vi "Load.vi"(8 "Error In":errorcluster, 10 "Key":string, 11 "Loader In":refnum<class "File.lvclass">) -> (0 "Error Out":errorcluster, 2 "Template":string, 3 "Loader Out":refnum<class "File.lvclass">)   [LabVIEW 2018, in "Toolkit.lvlib" / "Loaders.lvlib" / "File.lvclass"]
doc: "Gets a template as a string based on the Partial's key value in the root, or master, template.\n\n<B>Loader In/Out</B> - Represents an implementation capable of loading, or including, a partial Mustache template.\n\n<B>Key</B> - The key from the partial tag.\n\n<B>Template</B> - The partial Mustache template associated with the key. The origin of the template depends on the loader's implementation and the data type associated with the key."
uses:
  File.lvclass
  File.lvclass/File.ctl
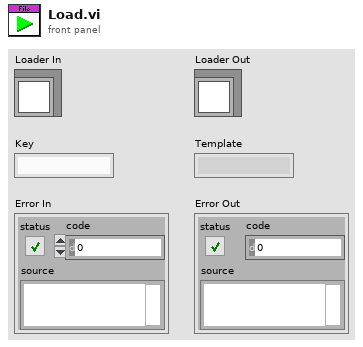
[diagram p1: front panel]
types:
  T1 = enum16{"open", "replace", "create", "open or create", "replace or create", "replace or create with confirmation"}
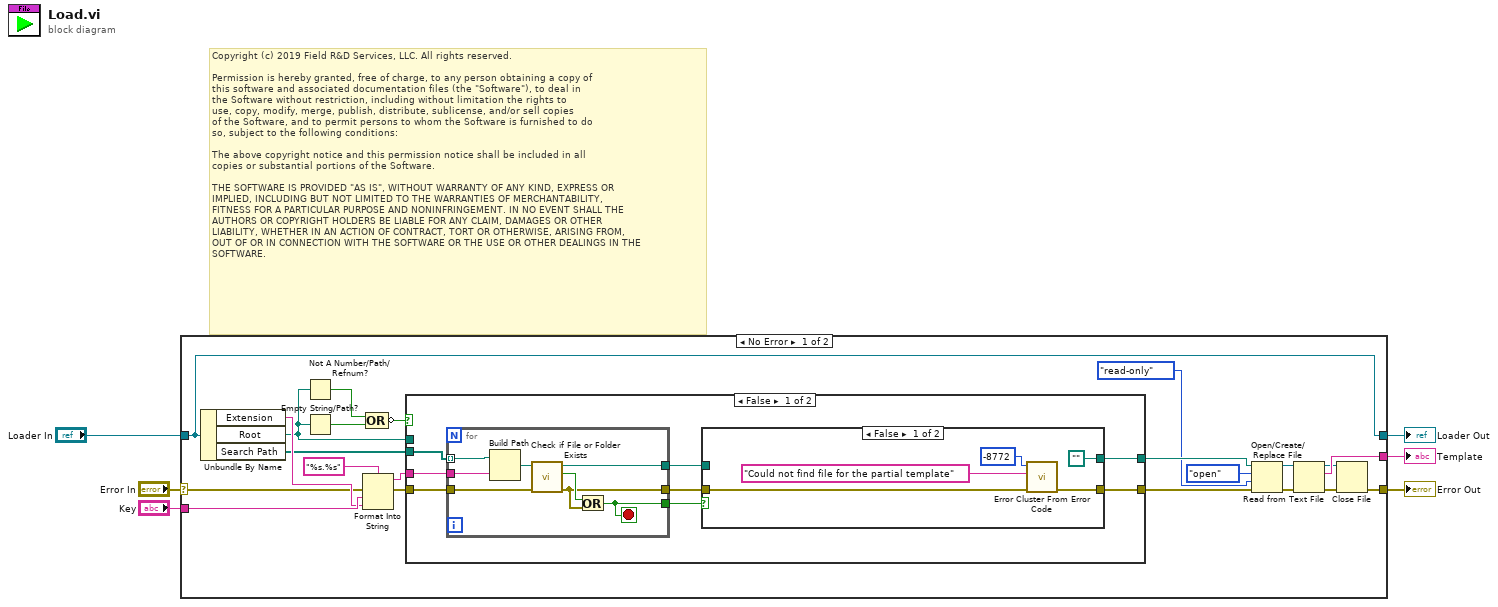
[diagram p0: block diagram]
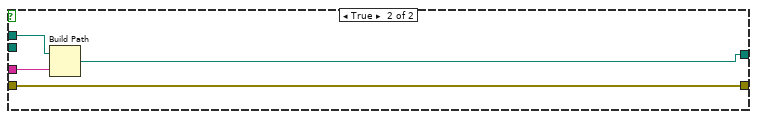
[diagram p3: hidden frame]
diagram:
  # "Copyright (c) 2019 Field R&D Services, LLC. All rights reserved.\n\nPermission is hereby granted, free of charge, to any person obtaining a copy of\nthis software and associated documentation files (the \"Software\"), to deal in\nthe Software without restriction, including without limitation the rights to\nuse, copy, modify, merge, publish, distribute, sublicense, and/or sell copies\nof the Software, and to permit persons to whom the Software is furnished to do\nso, subject to the following conditions:\n\nThe above copyright notice and this permission notice shall be included in all\ncopies or substantial portions of the Software.\n\nTHE SOFTWARE IS PROVIDED \"AS IS\", WITHOUT WARRANTY OF ANY KIND, EXPRESS OR\nIMPLIED, INCLUDING BUT NOT LIMITED TO THE WARRANTIES OF MERCHANTABILITY,\nFITNESS FOR A PARTICULAR PURPOSE AND NONINFRINGEMENT. IN NO EVENT SHALL THE\nAUTHORS OR COPYRIGHT HOLDERS BE LIABLE FOR ANY CLAIM, DAMAGES OR OTHER\nLIABILITY, WHETHER IN AN ACTION OF CONTRACT, TORT OR OTHERWISE, ARISING FROM,\nOUT OF OR IN CONNECTION WITH THE SOFTWARE OR THE USE OR OTHER DEALINGS IN THE\nSOFTWARE."
  n1 = case shown="No Error" "Error In" {
    selector: "Error In" -> [w25 w57]
    tunnel: [w16 w57] -> w5
    tunnel: "Loader In" -> [w15 w56]
    tunnel: [w15 w56] -> w3
    tunnel: "Key" -> [w28 _]
    tunnel: [w13 _] -> w1
    frame No Error {
      n2 = Unbundle By Name(w15) -> ("Extension"=w26:string, "Root"=w20:path, "Search Path"=w18:path[])
      n3 = Not A Number/Path/Refnum?(number/path/refnum=w20) -> (NaN/Path/Refnum?=w23:bool)
      n4 = Empty String/Path?(string/path=w20) -> (empty?=w24:bool)
      n5 = Format Into String(format string="%s.%s", error in=w25, w28, w26) -> (resulting string=w21:string, error out=w19:errorcluster)  [unwired: 1 in]
      n6 = Compound Arithmetic op=OR(w23, w24) -> (invert w22:bool)
      n7 = case shown="False" w22 {
        tunnel: w21 -> [w30 w55]
        tunnel: w20 -> [_ w54]
        tunnel: [w33 w53] -> w14
        tunnel: w19 -> [w36 w52]
        tunnel: [w31 w52] -> w17
        tunnel: w18 -> [w29 _]
        frame False {
          n8 = for {
            tunnel: w29 -> [w46] mode=indexing
            tunnel: w36 -> [w51]
            tunnel: [w49] -> w32
            tunnel: [w48] -> w34
            tunnel: [w47] -> w35
            tunnel: w30 -> [w45]
            stop <- w47 stop-if-true
            n9 = Build Path(base path=w46, name or relative path=w45) -> (appended path=w44:path)
            n10 = call <vilib>:"Check if File or Folder Exists.vi"("error in (no error)"=w51, "path"=w44) -> ("error out"=w49:errorcluster, "file or folder exists?"=w50:bool, "dup path"=w48:path)  [unwired: 7 in]
            n11 = Or(x=w50, y=w49) -> (x .or. y?=w47:bool)
          }
          n12 = case shown="False" w35 {
            tunnel: w34 -> [_ w43]
            tunnel: [path "" w43] -> w33
            tunnel: w32 -> [w40 w42]
            tunnel: [w39 w42] -> w31
            frame False {
              n13 = call <vilib>:"Error Cluster From Error Code.vi"("error in (no error)"=w40, "error message (\"\")"="Could not find file for the partial template" ("error message (\"\")"), "error code (0)"=-8772) -> ("error out"=w39:errorcluster)  [unwired: 6 in]
            }
            frame True {
            }
          }
        }
        frame True {
          n14 = Build Path(base path=w54, name or relative path=w55) -> (appended path=w53:path)
        }
      }
      n15 = Open/Create/Replace File(file path (use dialog)=w14, error in=w17, operation (0:open)=T1."open", access (0:read/write)=enum16{"read/write", "read-only", "write-only"}."read-only") -> (refnum out=w10:refnum<file>, error out=w9:errorcluster)  [unwired: 2 in, 1 out]
      n16 = Read from Text File(file (use dialog)=w10, error in=w9) -> (refnum out=w8:refnum<file>, text=w13:string, error out=w7:errorcluster)  [unwired: 2 in, 1 out]
      n17 = Close File(refnum=w8, error in=w7) -> (error out=w16:errorcluster)  [unwired: 1 out]
    }
    frame Error {
    }
  }
  "Loader Out" <- w3
  "Error Out" <- w5
  "Template" <- w1
